vi "VALEW_ATC_Verify Concurrent.vi"(0 "GEA2 Reference In":refnum<k24>, 11 "Error In":errorcluster) -> (4 "GEA2 Reference Out":refnum<k24>, 6 "Pass/fail?":bool, 8 "Report Text":string, 15 "Error Out":errorcluster)   [LabVIEW 2016, in "Centauro.lvlib"]
doc: "This test covers the ATC algorithm when doing a concurrent fill. A concurrent fill allows both hot and cold valves to be on at the same time. The valves are operated in parallel."
uses:
  Projects/Centauro.lvlib
  Q:/Common/DLLs/GEA3/GeaCommunication.dll
  Common/DLLs/GEA3/GeaCommunication.dll
  Common/LabVIEW GEA2 Toolkit/LabVIEW_GEA2_Toolkit.lvlibp/type defs/Source_Destination.ctl
  Common/LabVIEW GEA2 Toolkit/LabVIEW_GEA2_Toolkit.lvlibp/type defs/ERD Write Data In.ctl
  Common/LabVIEW GEA2 Toolkit/LabVIEW_GEA2_Toolkit.lvlibp/type defs/Data Type.ctl
  Common/LabVIEW GEA2 Toolkit/LabVIEW_GEA2_Toolkit.lvlibp/type defs/ERD Read Data In.ctl
  Valew Common/type defs/MC_Cycle_Engine_Request_State.ctl
  <vilib>/DAQmx/write.llb/DAQmx Write (Analog DBL 1Chan 1Samp).vi
  <vilib>/DAQmx/create/channels.llb/DAQmx Create Channel (AO-Voltage-Basic).vi
  <vilib>/DAQmx/miscellaneous.llb/DAQmx Fill In Error Info.vi
  Common/LabVIEW GEA2 Toolkit/LabVIEW_GEA2_Toolkit.lvlibp
panel:
  out "Valve time calculations pass?":bool
  out "Hot valve DAQ pass?":bool
  out "Cold valve DAQ pass?":bool
  out "Calc bath temp after seg gals":dbl
  out "Bath temp after seg gals":dbl
  out "Bath temp updated after segment fill?":bool
  in  "Standalone?":bool
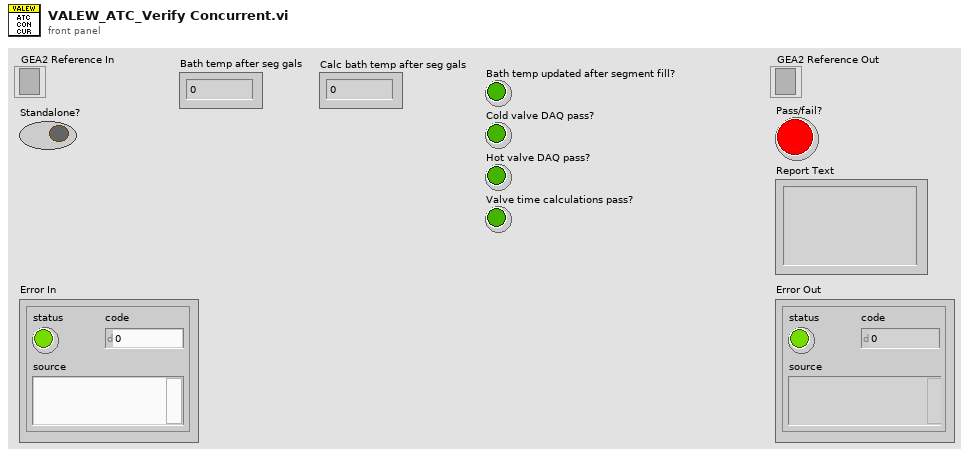
[diagram p1: front panel]
types:
  T1 = typedef "Centauro.lvlib/MC_Cycle_Engine_Request_State.ctl" = enum16{"Select", "Start", "Pause", "Resume", "Stop"}
  T2 = enum16{"EQ (==)", "NE (!=)", "GT (>)", "LT (<)", "GE (>=)", "LE (<=)", "GTLT(> <)", "GELE (>= <=)", "GELT (>= <)", "GTLE (> <=)", "LTGT (< >)", "LEGE (<= >=)", "LEGT (<= >)", "LTGE (< >=)", "No Comparison"}
  T3 = typedef "LabVIEW_GEA2_Toolkit.lvlibp/Source_Destination.ctl" = cluster{"Source":u8, "Destination":u8}
  T4 = typedef "LabVIEW_GEA2_Toolkit.lvlibp/ERD Read Data In.ctl" = cluster{"ERD Number":u16, "Data Type":T5}
  T5 = typedef "LabVIEW_GEA2_Toolkit.lvlibp/Data Type.ctl" = enum16{"string", "boolean", "uint8_t", "uint16_t", "uint32_t", "uint64_t", "int8_t", "int16_t", "int32_t", "int64_t"}
  T6 = typedef "LabVIEW_GEA2_Toolkit.lvlibp/ERD Write Data In.ctl" = cluster{"ERD Number":u16, "Data Type":T5, "Data":string}
  T7 = typedef "Centauro.lvlib/VALEW_ATC_Data.ctl" = cluster{"Accumulated hot gallons":dbl, "Accumulated cold gallons":dbl, "Current tub gallons":dbl, "Cold inlet temp (F)":dbl, "Hot inlet temp (F)":dbl, "Warm inlet temp (F)":dbl, "Hot valve time (s)":u16, "Cold valve time (s)":u16, "Current bath temp (F)":dbl, "Current water temp (F)":dbl, "Segment gallons":dbl}
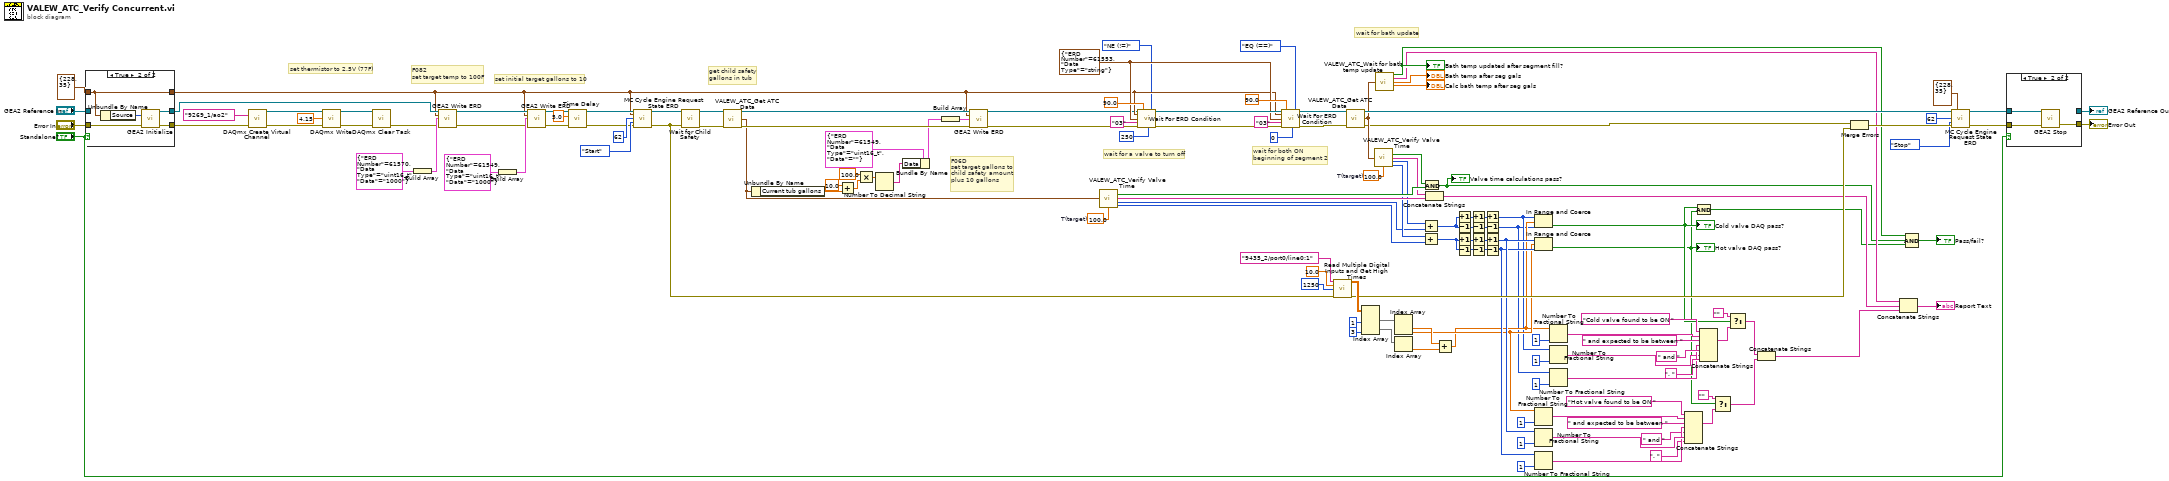
[diagram p0: block diagram]
diagram:
  w97 = 100.0  # T(target)
  w98 = 100.0  # T(target)
  w104 = T4 {"ERD Number"=61553, "Data Type"=enum."string"} ("ERD Read Data")
  # "set thermistor to 2.5V (77F)"
  # "wait for bath update"
  # "wait for both ON\nbeginning of segment 2"
  # "wait for a valve to turn off"
  # "set initial target gallons to 10"
  # "F06D\nset target gallons to\nchild safety amount\nplus 10 gallons"
  # "get child safety\ngallons in tub"
  # "F082\nset target temp to 100F"
  n1 = case shown="True" "Standalone?" {
    tunnel: T3 {"Source"=228, "Destination"=35} ("GEA Inputs") -> [w143 w146]
    tunnel: [w145 w149] -> w130
    tunnel: [w144 w148] -> w75
    tunnel: "Error In" -> [w144 w147]
    tunnel: "GEA2 Reference In" -> [w145 _]
    tunnel: [w143 w146] -> w72
    frame False {
    }
    frame True {
      n2 = Unbundle By Name(w146) -> ("Source"=w150:u8)
      n3 = call "GEA2 Initialize.vi"("Source Address"=w150, "error in"=w147) -> ("GEA2 Reference Out"=w149:refnum<k24>, "error out"=w148:errorcluster)  [unwired: 11 in, 1 out]
    }
  }
  n4 = call-poly <vilib>:"DAQmx Create Virtual Channel.vi"("physical channels"=tag "9269_1/ao2", "error in"=w75) -> ("task out"=w80:refnum<k21>, "error out"=w74:errorcluster)  [unwired: 12 in]
  n5 = call-poly <vilib>:"DAQmx Write.vi"("task/channels in"=w80, "data"=4.15, "error in"=w74) -> ("task out"=w76:refnum<k21>, "error out"=w77:errorcluster)  [unwired: 10 in, 1 out]
  n6 = call <vilib>:"DAQmx Clear Task.vi"("task in"=w76, "error in"=w77) -> ("error out"=w73:errorcluster)  [unwired: 13 in]
  n7 = Build Array(T6 {"ERD Number"=61570, "Data Type"=enum."uint16_t", "Data"="1000"} ("ERD Write Data In")) -> (w137:T6[])
  n8 = call "GEA2 Write ERD.vi"("GEA2 Reference In"=w130, "GEA Inputs"=w72, "Write ERD List"=w137, "Error In"=w73) -> ("GEA2 Reference Out"=w119:refnum<k24>, "Error Out"=w118:errorcluster)  [unwired: 9 in, 1 out]
  n9 = Build Array(T6 {"ERD Number"=61549, "Data Type"=enum."uint16_t", "Data"="1000"} ("ERD Write Data In")) -> (w120:T6[])
  n10 = call "GEA2 Write ERD.vi"("GEA2 Reference In"=w119, "GEA Inputs"=w72, "Write ERD List"=w120, "Error In"=w118) -> ("GEA2 Reference Out"=w117:refnum<k24>, "Error Out"=w2:errorcluster)  [unwired: 9 in, 1 out]
  n11 = call "Time Delay"("error in (no error)"=w2, "Delay Time (s)"=5.0) -> ("error out"=w1:errorcluster)  [unwired: 9 in]
  n12 = call "MC Cycle Engine Request State ERD.vi"("GEA2 Reference In"=w117, "GEA Inputs"=w72, "Cycle #"=u8 62, "MC Cycle Engine State"=MC_Cycle_Engine_Request_State."Start", "Error In"=w1) -> ("GEA2 Reference Out"=w139:refnum<k24>, "Error Out"=w70:errorcluster)  [unwired: 9 in]
  n13 = call "Wait for Child Safety.vi"("GEA2 Reference In"=w139, "Error In"=w70) -> ("GEA2 Reference Out"=w92:refnum<k24>, "Error Out"=w85:errorcluster)  [unwired: 9 in, 3 out]
  n14 = call "VALEW_ATC_Get ATC Data.vi"("GEA2 Reference In"=w92, "Error In"=w85) -> ("GEA2 Reference Out"=w128:refnum<k24>, "ATC Data"=w8:T7, "Error Out"=w129:errorcluster)  [unwired: 11 in]
  n15 = Unbundle By Name(w8) -> ("Current tub gallons"=w103:dbl)
  n16 = Add(x=10.0, y=w103) -> (x+y=w123:dbl)
  n17 = Multiply(x=100.0, y=w123) -> (x*y=w124:dbl)
  n18 = Number To Decimal String(number=w124) -> (decimal integer string=w116:string)  [unwired: 1 in]
  n19 = Bundle By Name(cluster=T6 {"ERD Number"=61549, "Data Type"=enum."uint16_t", "Data"=""} ("ERD Write Data In"), "Data"=w116) -> (w125:T6)
  n20 = Build Array(w125) -> (w136:T6[])
  n21 = call "GEA2 Write ERD.vi"("GEA2 Reference In"=w128, "GEA Inputs"=w72, "Write ERD List"=w136, "Error In"=w129) -> ("GEA2 Reference Out"=w6:refnum<k24>, "Error Out"=w7:errorcluster)  [unwired: 9 in, 1 out]
  n22 = call "VALEW_ATC_Verify Valve Time.vi"("ATC Data"=w8, "T(target)"=w98) -> ("Pass/Fail?"=w95:bool, "Report Text"=w93:string, "Cold valve time (s) ATC"=w82:u16, "Hot valve time (s) ATC"=w81:u16)  [unwired: 10 in]
  n23 = call "Wait For ERD Condition.vi"("GEA2 Reference In"=w6, "GEA Inputs"=w72, "ERD Read Data"=w104, "Expected Low"="03", "Error In"=w7, "Timeout (s)"=90.0, "Loop Rate (ms)"=u32 250, "Comparison"=T2."NE (!=)") -> ("GEA2 Reference Out"=w115:refnum<k24>, "Error Out"=w114:errorcluster)  [unwired: 7 in, 3 out]
  n24 = call "Wait For ERD Condition.vi"("GEA2 Reference In"=w115, "GEA Inputs"=w72, "ERD Read Data"=w104, "Expected Low"="03", "Error In"=w114, "Timeout (s)"=90.0, "Loop Rate (ms)"=u32 0, "Comparison"=T2."EQ (==)") -> ("GEA2 Reference Out"=w100:refnum<k24>, "Error Out"=w101:errorcluster)  [unwired: 7 in, 3 out]
  n25 = call "Read Multiple Digital Inputs and Get High Times.vi"("Lines"=tag "9435_2/port0/line0:1", "Rate (Hz)"=10.0 ("rate"), "Samples"=1250 ("samples per channel"), "Error In"=w70) -> ("High Times (s)"=w88:dbl[][], "Error Out"=w54:errorcluster)  [unwired: 10 in]
  n26 = call "VALEW_ATC_Get ATC Data.vi"("GEA2 Reference In"=w100, "Error In"=w101) -> ("GEA2 Reference Out"=w102:refnum<k24>, "ATC Data"=w71:T7, "Error Out"=w53:errorcluster)  [unwired: 11 in]
  n27 = Index Array(array=w88, index (col) #1=1 ("disabled index (col)"), index (col) #2=3 ("index (col)")) -> (element #1=w86:dbl[], element #2=w59:dbl[])  [unwired: 2 in]
  n28 = call "VALEW_ATC_Verify Valve Time.vi"("ATC Data"=w71, "T(target)"=w97) -> ("Pass/Fail?"=w96:bool, "Report Text"=w94:string, "Cold valve time (s) ATC"=w84:u16, "Hot valve time (s) ATC"=w83:u16)  [unwired: 10 in]
  n29 = call "VALEW_ATC_Wait for bath temp update.vi"("ATC Data"=w71) -> ("Bath temp updated after segment fill?"=w51:bool, "Report Text"=w48:string, "Bath temp after seg gals"=→"Bath temp after seg gals":dbl, "Calc bath temp after seg gals"=→"Calc bath temp after seg gals":dbl)  [unwired: 11 in]
  "Bath temp updated after segment fill?" <- w51
  n30 = Index Array(array=w86) -> (element #1=w57:dbl, element #2=w33:dbl)  [unwired: 2 in]
  n31 = Index Array(array=w59) -> (element=w58:dbl)  [unwired: 1 in]
  n32 = Add(x=w84, y=w82) -> (x+y=w62:u16)
  n33 = Add(x=w83, y=w81) -> (x+y=w61:u16)
  n34 = And(x=w96, y=w95) -> (x .and. y?=w13:bool)
  "Valve time calculations pass?" <- w13
  n35 = Concatenate Strings(w94, w93) -> (w12:string)
  n36 = Add(x=w57, y=w58) -> (x+y=w20:dbl)
  n37 = Increment(x=w62) -> (x+1=w66:u16)
  n38 = Decrement(x=w62) -> (x-1=w69:u16)
  n39 = Increment(x=w61) -> (x+1=w68:u16)
  n40 = Decrement(x=w61) -> (x-1=w67:u16)
  n41 = Increment(x=w66) -> ()  [unwired: 1 out]
  n42 = Decrement(x=w69) -> (x-1=w65:u16)
  n43 = Increment(x=w68) -> (x+1=w64:u16)
  n44 = Decrement(x=w67) -> (x-1=w63:u16)
  n45 = Increment(x=w66) -> (x+1=w19:u16)
  n46 = Decrement(x=w65) -> (x-1=w18:u16)
  n47 = Increment(x=w64) -> (x+1=w36:u16)
  n48 = Decrement(x=w63) -> (x-1=w35:u16)
  n49 = In Range and Coerce(upper limit=w19, x=w20, lower limit=w18) -> (In Range?=w15:bool)  [unwired: 1 out]
  "Cold valve DAQ pass?" <- w15
  n50 = In Range and Coerce(upper limit=w36, x=w33, lower limit=w35) -> (In Range?=w14:bool)  [unwired: 1 out]
  "Hot valve DAQ pass?" <- w14
  n51 = Number To Fractional String(number=w33, precision (6)=i16 1) -> (F-format string=w42:string)  [unwired: 2 in]
  n52 = Number To Fractional String(number=w36, precision (6)=i16 1) -> (F-format string=w47:string)  [unwired: 2 in]
  n53 = Number To Fractional String(number=w35, precision (6)=i16 1) -> (F-format string=w40:string)  [unwired: 2 in]
  n54 = Number To Fractional String(number=w20, precision (6)=i16 1) -> (F-format string=w26:string)  [unwired: 2 in]
  n55 = Number To Fractional String(number=w19, precision (6)=i16 1) -> (F-format string=w21:string)  [unwired: 2 in]
  n56 = Number To Fractional String(number=w18, precision (6)=i16 1) -> (F-format string=w28:string)  [unwired: 2 in]
  n57 = Concatenate Strings("Hot valve found to be ON ", w42, " and expected to be between ", w40, " and " ("string"), w47, ". " ("string")) -> (w37:string)
  n58 = Compound Arithmetic op=AND(w15, w14) -> (w11:bool)
  n59 = Concatenate Strings("Cold valve found to be ON ", w26, " and expected to be between ", w28, " and " ("string"), w21, ". " ("string")) -> (w31:string)
  n60 = Select(t="", s=w14, f=w37) -> (s? t:f=w16:string)
  n61 = Select(t="", s=w15, f=w31) -> (s? t:f=w17:string)
  n62 = Concatenate Strings(w17, w16) -> (w10:string)
  n63 = Merge Errors(w53, w54) -> (w52:errorcluster)
  n64 = Concatenate Strings(w48, w12, w10) -> (→"Report Text":string)
  n65 = Compound Arithmetic op=AND(w51, w13, w11) -> (→"Pass/fail?":bool)
  n66 = call "MC Cycle Engine Request State ERD.vi"("GEA2 Reference In"=w102, "GEA Inputs"=T3 {"Source"=228, "Destination"=35}, "Cycle #"=u8 62, "MC Cycle Engine State"=MC_Cycle_Engine_Request_State."Stop", "Error In"=w52) -> ("GEA2 Reference Out"=w131:refnum<k24>, "Error Out"=w132:errorcluster)  [unwired: 9 in]
  n67 = case shown="True" "Standalone?" {
    tunnel: w132 -> [w152 w155]
    tunnel: w131 -> [w151 w154]
    tunnel: [w152 w153] -> w134
    tunnel: [w151 _] -> w135
    frame False {
    }
    frame True {
      n68 = call "GEA2 Stop.vi"("GEA2 Reference In"=w154, "Error In"=w155) -> ("Error Out"=w153:errorcluster)  [unwired: 13 in]
    }
  }
  "GEA2 Reference Out" <- w135
  "Error Out" <- w134
